vi "picoGet.vi"(8 "error in (no error)":errorcluster, 9 "postTriggerSamples":u32, 10 "Rapid Block Acquisition Settings":T1, 11 "Handle In":i16) -> (0 "error out":errorcluster, 2 "buffer":i16[][](array[numeric]), 3 "handle":i16)   [LabVIEW 2011]
uses:
  PS2000a.dll
panel:
  in  "nCaptures":u16
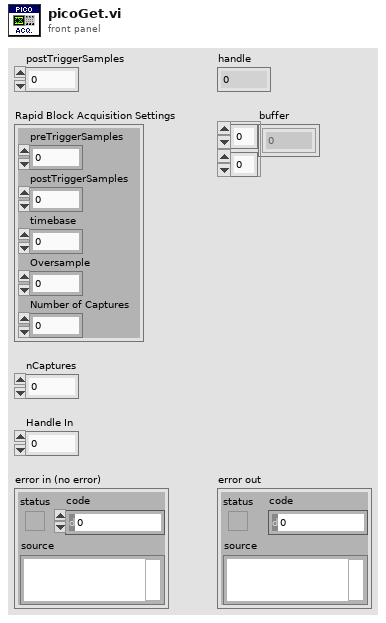
[diagram p1: front panel]
types:
  T1 = cluster{"preTriggerSamples":u32, "postTriggerSamples":u32, "timebase":u32, "Oversample":i16, "Number of Captures":u32}
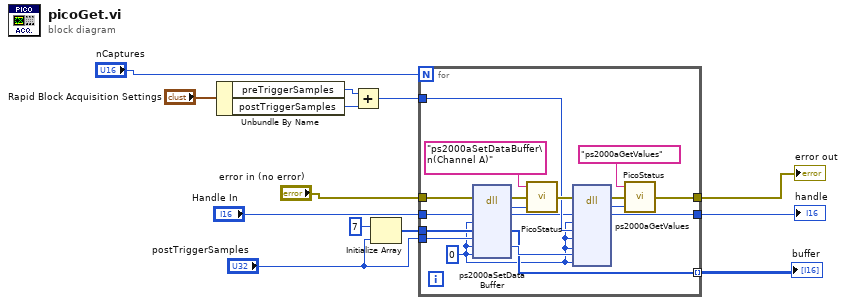
[diagram p0: block diagram]
diagram:
  n1 = Unbundle By Name("Rapid Block Acquisition Settings") -> ("preTriggerSamples"=w4:u32, "postTriggerSamples"=w3:u32)
  n2 = Add(x=w4, y=w3) -> (x+y=w5:u32)
  n3 = Initialize Array(i16 7 ("element"), "postTriggerSamples") -> (w9:i16[])
  n4 = for {
    N: "nCaptures" -> [_]
    tunnel: "error in (no error)" -> [w28]
    tunnel: "Handle In" -> [w27]
    tunnel: "postTriggerSamples" -> [w26]
    tunnel: w5 -> [w21]
    tunnel: [w19] -> w6
    tunnel: [w18] -> w7
    tunnel: w9 -> [w16]
    tunnel: [w15] -> w10 mode=indexing
    w14 = 0 ("channel")
    n5 = dll-call lib="ps2000a.dll" fn="ps2000aSetDataBuffer" ("ps3000.dll:_ps3000_open_unit@0")(error in=w28, "handle"=w27, "channel"=w14, "buffer"=w16, "bufferLth"=w26, "waveform"=w14, "downSampleRatioMode"=w14) -> (error out=w30:errorcluster, "PICO_STATUS"=w31:i32, "handle"=w20:i16, "buffer"=w15:i16[], "waveform"=w17:u32)  [unwired: 5 in, 1 out]
    n6 = call "PicoStatus.vi"("PICO STATUS"=w31, "error in"=w30, "source"="ps2000aSetDataBuffer\n(Channel A)") -> ("error out"=w22:errorcluster)
    n7 = dll-call lib="ps2000a.dll" fn="ps2000aGetValues" ("ps3000.dll:_ps3000_open_unit@0")(error in=w22, "handle"=w20, "startIndex"=w14, "noOfSamples"=w21, "downSampleRatio"=w14, "downSampleRatioMode"=w14, "segmentIndex"=w17, "overflow"=w14) -> (error out=w24:errorcluster, "PICO_STATUS"=w25:i32, "handle"=w19:i16)  [unwired: 8 in, 1 out]
    n8 = call "PicoStatus.vi"("PICO STATUS"=w25, "error in"=w24, "source"="ps2000aGetValues") -> ("error out"=w18:errorcluster)
  }
  "buffer" <- w10
  "error out" <- w7
  "handle" <- w6
